vi "1.Main demo.vi"() -> ()   [LabVIEW 2015]
uses:
  UnderAutomation.Fanuc/UnderAutomation.Fanuc.lvlib
  C:/Users/fg/Documents/Fanuc.vi/LabVIEW_2024/UnderAutomation.Fanuc/lib/UnderAutomation.Fanuc.dll
  LabVIEW_2024/UnderAutomation.Fanuc/lib/UnderAutomation.Fanuc.dll
panel:
  out "CGTP Enabled":bool
  out "Cgtp":refnum<k24>
  out "SNPX connected":bool
  out "FTP connected":bool
  out "Telnet connected":bool
  in  "Tab Control":T1(tab)
  in  "HTTP Password":string caption="HTTP password"
  in  "HTTP Login":string caption="HTTP login (optional)"
  in  "Use CGTP":bool
  in  "Disconnect":bool
  in  "Test":bool
  in  "Key":string
  in  "Licensee":string
  in  "Use SNPX":bool
  in  "FTP password":string
  in  "FTP user":string
  in  "Use FTP":bool
  in  "Connect":bool
  in  "Telnet password":string
  in  "Use Telnet":bool
  in  "ConnectRoboguide":bool
  in  "RoboguideRobotPath":path caption="Path to \"Robot\" ROBOGUIDE folder that contains services.txt"
  in  "IP":string caption="Robot IP Address"
  out "License state":string
  out "Connect error":string
  out "CGTP warning":string
  in  "Abort":bool
  in  "Pause":bool
  in  "Program name":string caption="Program name without extension"
  in  "Run":bool
  in  "Write variable as real":bool
  in  "New integer value":i32
  in  "New real value":dbl
  in  "String value":string
  in  "Variable name":string
  in  "Write variable as integer":bool
  in  "Read variable":bool
  in  "Write variable as string":bool
  in  "Unsimulate all":bool
  in  "Unsimulate":bool
  in  "Simulate":bool
  in  "Set port value":bool
  in  "Variable set value":bool
  in  "Variable new value":string caption="New value"
  in  "Variable get value":bool
  in  "Variable name":string
  out "Telnet warning":string
  out "Current position":T2
  in  "Get current position":bool
  in  "Reset alarms":bool
  in  "Get task info":bool
  in  "Task name":string caption="Task name (program without extension)"
  in  "Abort all programs":bool
  in  "Clear variable":bool
  in  "Clear Program":bool
  in  "Hold":bool
  in  "Continue":bool
  in  "Abort":bool
  in  "Pause":bool
  in  "Program name":string caption="Program name without extension"
  in  "Run":bool
  out "TelnetError":string caption="Error :"
  out "TelnetSucceed":bool caption="Succeeded"
  out "KclCommand":string caption="Last command :"
  out "TaskInfo":T3
  out "Variable value":string
  in  "port":i32(ring) items=["DIN", "DOUT", "RDO", "OPOUT", "TPOUT", "WDI", "WDO", "AIN", "AOUT", "GIN", "GOUT"]
  in  "index":i32
  in  "value":i32
  out "FTP warning":string
  out "PosReg":T4(array[cluster])
  out "StrReg":string[](array[string])
  in  "Tab Control IO state":T5(tab)
  out "UI":cluster{"Id":i32, "Name":string, "Value":bool}[](array[cluster])
  out "UO":cluster{"Id":i32, "Name":string, "Value":bool}[](array[cluster])
  out "SI":cluster{"Id":i32, "Name":string, "Value":bool}[](array[cluster])
  out "SO":cluster{"Id":i32, "Name":string, "Value":bool}[](array[cluster])
  out "DIN":cluster{"Id":i32, "Name":string, "Value":bool}[](array[cluster])
  out "DOUT":cluster{"Id":i32, "Name":string, "Value":bool}[](array[cluster])
  out "RI":cluster{"Id":i32, "Name":string, "Value":bool}[](array[cluster])
  out "RO":cluster{"Id":i32, "Name":string, "Value":bool}[](array[cluster])
  out "FLG":cluster{"Id":i32, "Name":string, "Value":bool}[](array[cluster])
  in  "Tab Control position":enum32{"World", "Joints", "User frames"}(tab)
  out "World Positions":T6(array[cluster])
  out "JointsPosition":dbl[](array[numeric])
  out "UserFramePositions":T7(array[cluster])
  in  "Get current position":bool
  in  "Get IO State":bool
  in  "Port":i32(ring) items=["DIN", "DOUT", "UI", "UO", "SI", "SO", "RI", "RO", "FLG"]
  out "Errors":T8(array[cluster])
  in  "Get all errors":bool
  in  "Get safety status":bool
  out "SafetyStatus":T9
  out "NumReg":dbl[](array[numeric])
  in  "Get numeric registers":bool
  in  "Get string registers":bool
  in  "Get position registers":bool
  out "SNPX warning":string
  in  "Tab Control snpx register":enum32{"Cartesian", "Joints"}(tab)
  in  "Cartesian position 2":T10
  in  "Write cartesian position register":bool
  in  "Joints position":dbl[](array[numeric])
  in  "Write joints position register":bool
  in  "Position register":i32
  in  "Read position register":bool
  out "Value":string
  in  "New value":string
  in  "String register":i32
  in  "Read string register":bool
  in  "Write string register":bool
  in  "Continuous read world position":bool
  out "JointsPosition":dbl[](array[numeric])
  out "Cartesian position":T11
  out "UserTool":i16
  out "error out":errorcluster
  in  "Continuous read user frame position":bool
  in  "userFrame":i32
  out "Cartesian position":T11
  out "UserTool":i16
  out "error out 2":errorcluster
  in  "Numeric register":i32
  in  "New value":sgl
  out "Value":sgl
  in  "Read numeric register":bool
  in  "Write numeric register":bool
  out "UserFrame":i16
  out "UserTool":i16
  in  "stop":bool
  out "Snpx":refnum<k24>
  out "Ftp":refnum<k24>
  out "Telnet":refnum<k24>
  out "robot":refnum<k24>
  # "UnderAutomation"
  # "https://underautomation.com/fanuc"
  # "+"
  # "LabVIEW demo app for remote control and monitoring of your Fanuc robot"
  # "Connect to robot"
  # "2. Ensure you have a trial or lifetime valid license"
  # "1. Set Fanuc robot address"
  # "This is a commercial library, you have a 30-day trial period. But you can use it forever if you buy a perpetual licence for your company (regardless of the number of robot, applications or developers)."
  # "Connect to real robot"
  # "Connect to ROBOGUIDE"
  # "If you have a license :"
  # "3. Select the services you want to connect to"
  # "CGTP"
  # "Telnet"
  # "FTP"
  # "SNPX"
  # "You need option R553 \"HMI Device SNPX\" \nor R651 FRL"
  # "How to enable Telnet : https://underautomation.com/fanuc/documentation/enable-telnet"
  # "See : https://underautomation.com/fanuc/documentation/snpx"
  # "4. Connect to the robot"
  # "CGTP"
  # "Please note that other CGTP features are available and can be provided upon request. Please contact UnderAutomation."
  # "Program execution"
  # "Variable"
  # "Telnet"
  # "Variables"
  # "Program execution"
  # "Task"
  # "Ports"
  # "Current position"
  # "Alarms"
  # "FTP"
  # "Current Position"
  # "IO State"
  # "Errors"
  # "Registers"
  # "Safety status"
  # "SNPX"
  # "Numeric registers"
  # "String registers"
  # "Read world position"
  # "Read user frame position"
  # "Position registers"
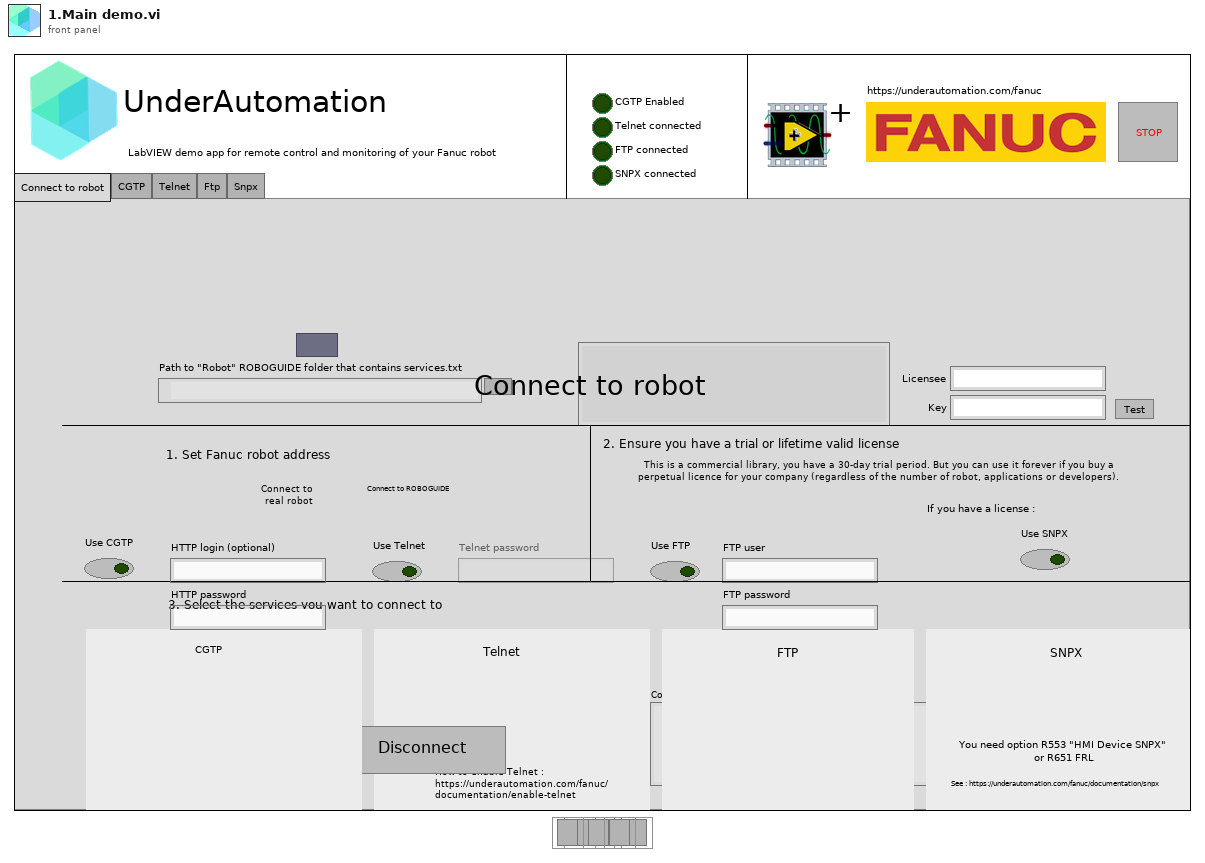
[diagram p1: front panel]
types:
  T1 = enum32{"Connect to robot", "CGTP", "Telnet", "Ftp", "Snpx"}
  T2 = cluster{"X":dbl, "Y":dbl, "Z":dbl, "W":dbl, "P":dbl, "R":dbl}
  T3 = cluster{"CurrentLine":i32, "RoutineName":string, "SystemTask":bool, "TaskName":string, "TaskNumber":i32, "TaskStatus":i32, "TaskStatusStr":string}
  T4 = cluster{"X":dbl, "Y":dbl, "Z":dbl, "W":dbl, "P":dbl, "R":dbl}[][]
  T5 = enum32{"UI", "UO", "SI", "SO", "DIN", "DOUT", "RI", "RO", "FLG"}
  T6 = cluster{"Tool":i32, "Cartesian position":cluster{cluster{"ArmFrontBack":i32, "ArmLeftRight":i32, "ArmUpDown":i32, "TurnAxis1":i32, "TurnAxis2":i32, "TurnAxis3":i32, "WristFlip":i32}, "X":dbl, "Y":dbl, "Z":dbl, "W":dbl, "P":dbl, "R":dbl}}[]
  T7 = cluster{"Frame":i32, "Tool":i32, "Cartesian position":cluster{cluster{"ArmFrontBack":i32, "ArmLeftRight":i32, "ArmUpDown":i32, "TurnAxis1":i32, "TurnAxis2":i32, "TurnAxis3":i32, "WristFlip":i32}, "X":dbl, "Y":dbl, "Z":dbl, "W":dbl, "P":dbl, "R":dbl}}[]
  T8 = cluster{"Id":i32, "IsReset":bool, "Text":string}[]
  T9 = cluster{"BeltBroken":bool, "ExternalEStop":bool, "FenceOpen":bool, "HandBroken":bool, "LowAirAlarm":bool, "NonTeacherEnb":bool, "OverTravel":bool, "SOPEStop":bool, "SVOFFDetect":bool, "TPDeadman":bool, "TPEnable":bool, "TPEStop":bool}
  T10 = cluster{"Configuration":cluster{"ArmFrontBack":i32, "ArmLeftRight":i32, "ArmUpDown":i32, "TurnAxis1":i32, "TurnAxis2":i32, "TurnAxis3":i32, "WristFlip":i32}, "X":dbl, "Y":dbl, "Z":dbl, "W":dbl, "P":dbl, "R":dbl}
  T11 = cluster{"Cartesian position":cluster{cluster{"ArmFrontBack":i32, "ArmLeftRight":i32, "ArmUpDown":i32, "TurnAxis1":i32, "TurnAxis2":i32, "TurnAxis3":i32, "WristFlip":i32}, "X":dbl, "Y":dbl, "Z":dbl, "W":dbl, "P":dbl, "R":dbl}, "Extension":cluster{"E1":dbl, "E2":dbl, "E3":dbl, "T4":i16, "T5":i16, "T6":i16}}
  T12 = enum8{"Enabled", "Disabled", "Disabled and Grayed Out"}
  T13 = cluster{"Id":i32, "Values":dbl[], "UserFramePositions":cluster{"Frame":i32, "Tool":i32, "Cartesian position":cluster{cluster{"ArmFrontBack":i32, "ArmLeftRight":i32, "ArmUpDown":i32, "TurnAxis1":i32, "TurnAxis2":i32, "TurnAxis3":i32, "WristFlip":i32}, "X":dbl, "Y":dbl, "Z":dbl, "W":dbl, "P":dbl, "R":dbl}}[], "World Positions":cluster{"Tool":i32, "Cartesian position":cluster{cluster{"ArmFrontBack":i32, "ArmLeftRight":i32, "ArmUpDown":i32, "TurnAxis1":i32, "TurnAxis2":i32, "TurnAxis3":i32, "WristFlip":i32}, "X":dbl, "Y":dbl, "Z":dbl, "W":dbl, "P":dbl, "R":dbl}}[]}[]
  T14 = cluster{"Id":i32, "Name":string, "Port":i32, "Value":bool, "PortStr":string}[]
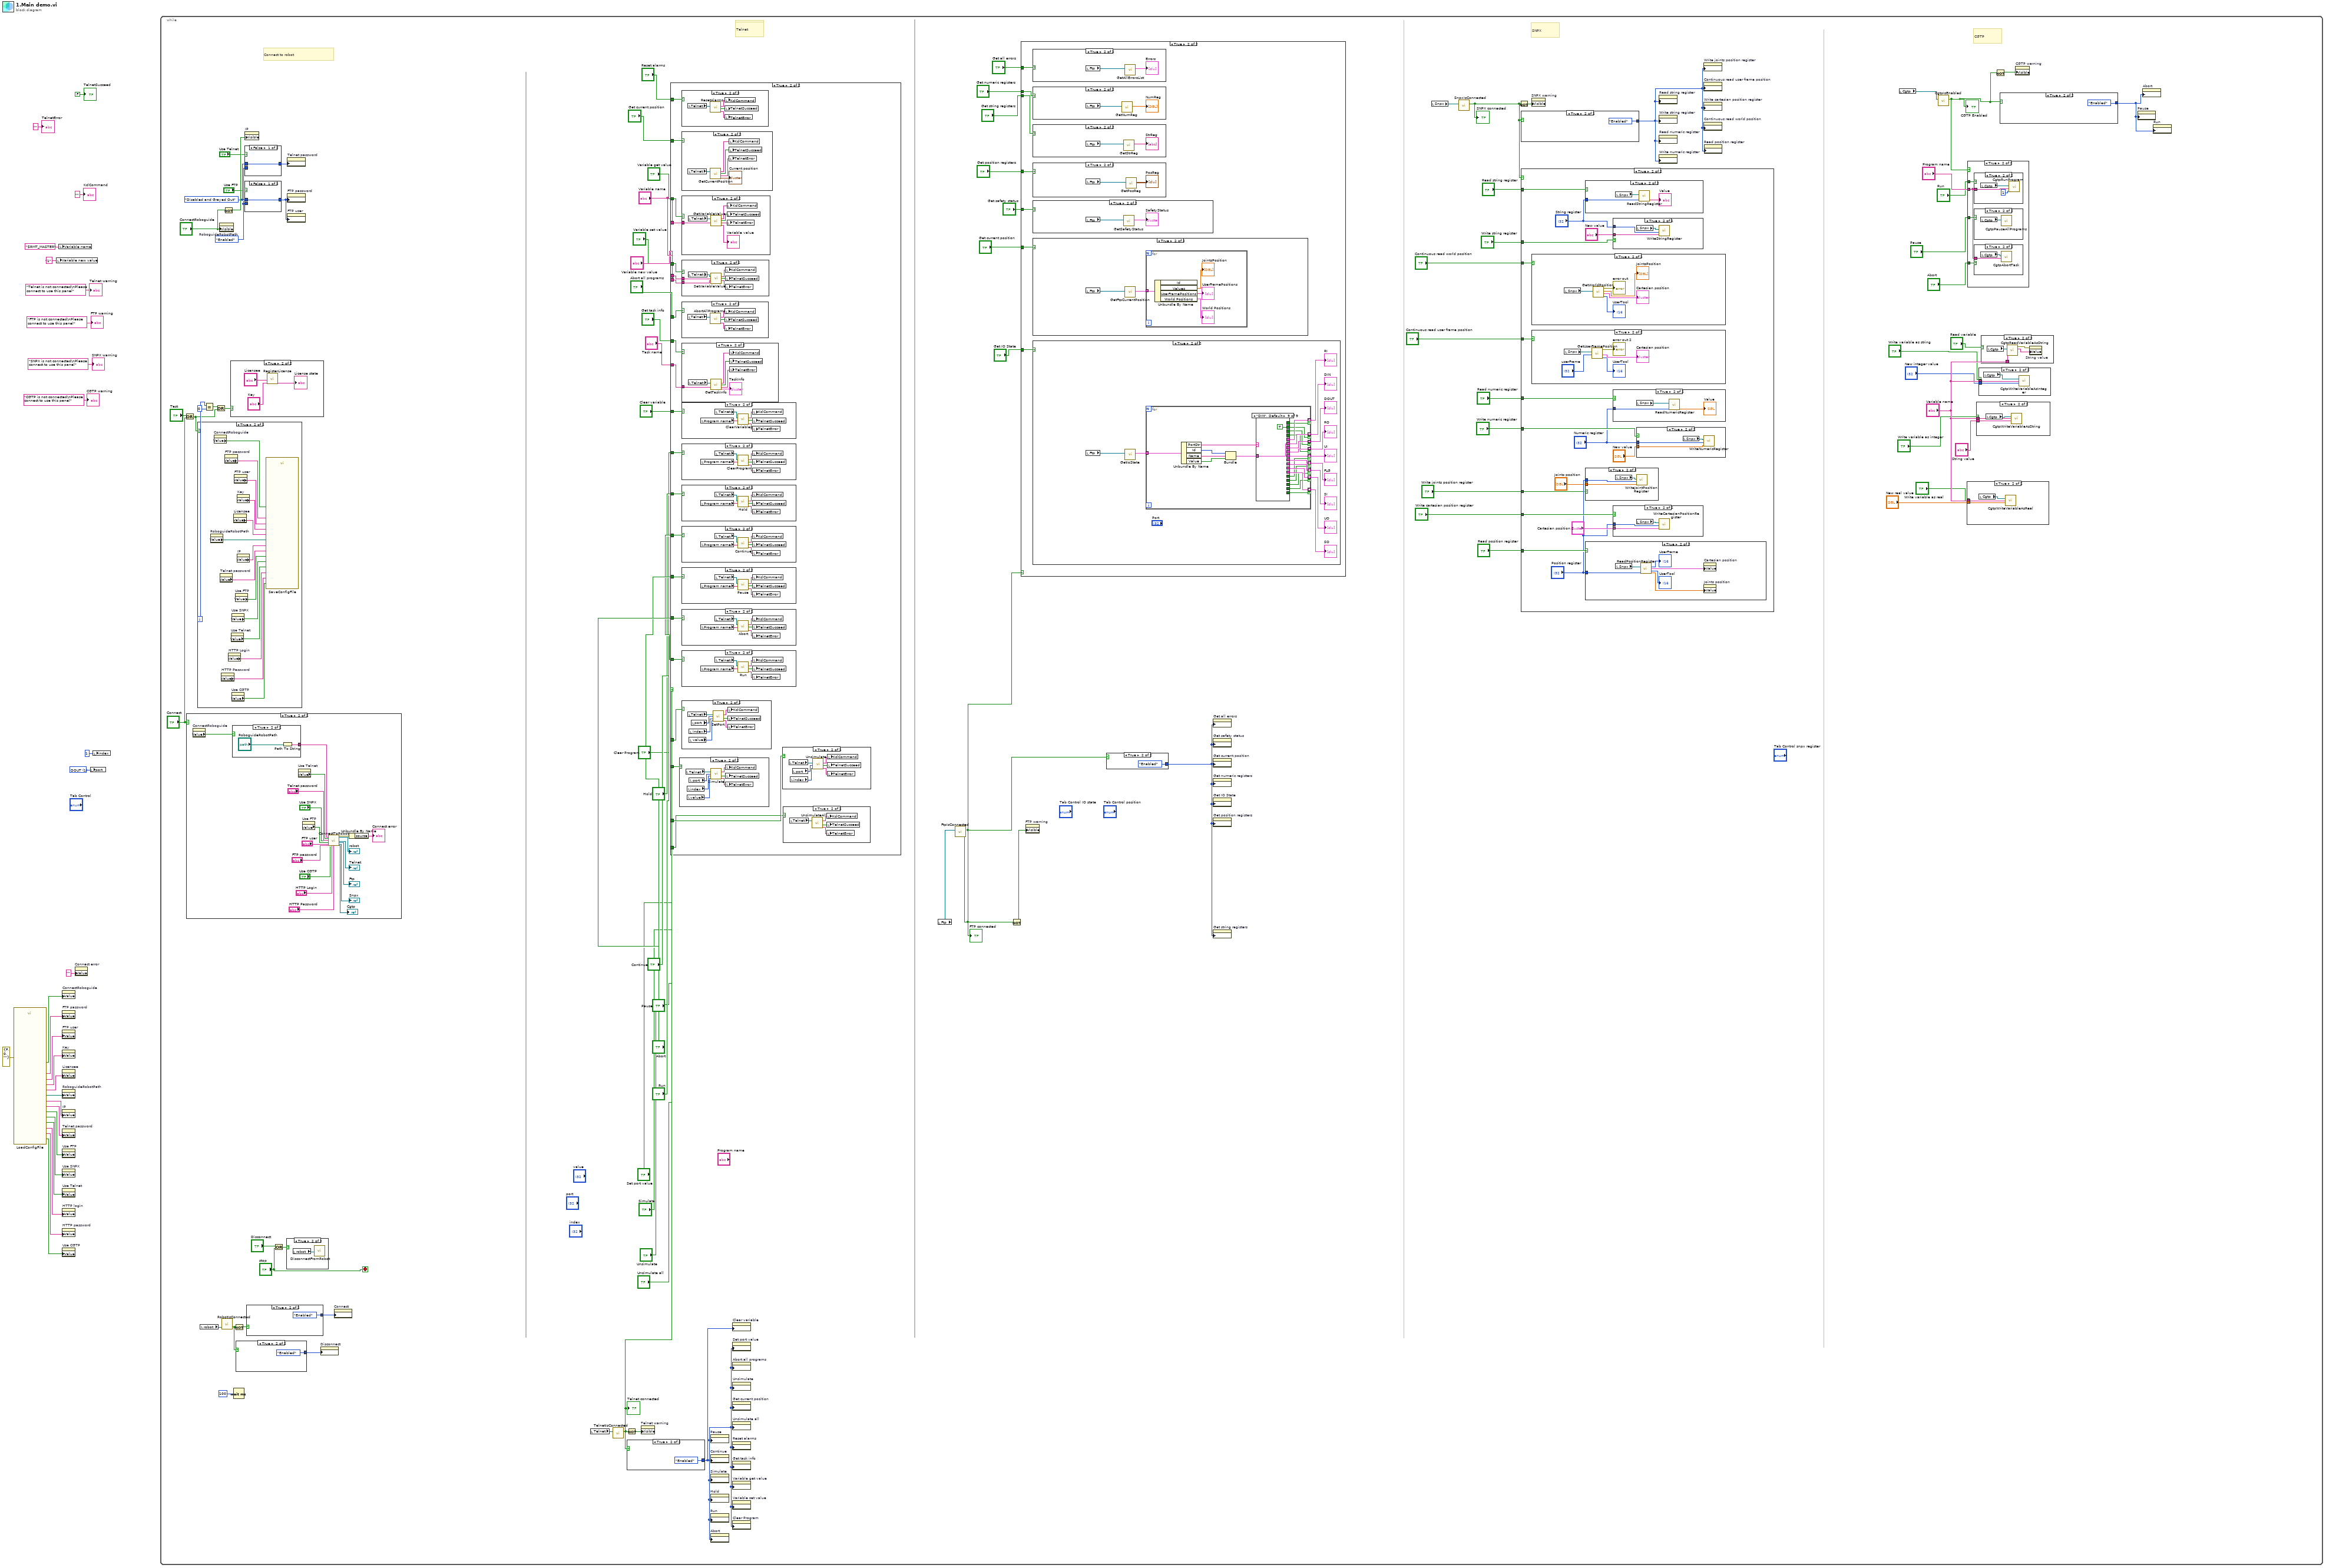
[diagram p0: block diagram]
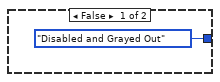
[diagram p10: hidden frame]
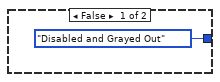
[diagram p11: hidden frame]
diagram:
  w7 = 1 items=["DIN", "DOUT", "RDO", "OPOUT", "TPOUT", "WDI", "WDO", "AIN", "AOUT", "GIN", "GOUT"] ("port")
  n1 = call "LoadConfigFile.vi"("error in (no error)"=errorcluster {"status"=FALSE, "code"=0, "source"=""}) -> ("Use CGTP"=w2:bool, "HTTP login"=w3:string, "HTTP password"=w4:string, "FTP password"=w24:string, "Licensee"=w16:string, "FTP user"=w23:string, "Key"=w17:string, "Use FTP"=w20:bool, "IP"=w26:string, "RoboguideRobotPath"=w22:path, "ConnectRoboguide"=w25:bool, "Use Telnet"=w18:bool, "Telnet password"=w21:string, "Use SNPX"=w19:bool)  [unwired: 12 in, 1 out]
  n2 = local write "Variable new value"("1" ("Variable new value")) -> ()
  n3 = local write "Variable name"("$RMT_MASTER" ("Variable name")) -> ()
  n4 = property on="ConnectRoboguide" class="Bool (strict)"("Value"=w25) -> ()  [unwired: 2 in, 2 out]
  n5 = property on="FTP password" class="Str"("Value"=w24) -> ()  [unwired: 2 in, 2 out]
  n6 = property on="FTP user" class="Str"("Value"=w23) -> ()  [unwired: 2 in, 2 out]
  n7 = property on="Key" class="Str"("Value"=w17) -> ()  [unwired: 2 in, 2 out]
  n8 = property on="Licensee" class="Str"("Value"=w16) -> ()  [unwired: 2 in, 2 out]
  n9 = property on="RoboguideRobotPath" class="Path"("Value"=w22) -> ()  [unwired: 2 in, 2 out]
  n10 = property on="IP" class="Str"("Value"=w26) -> ()  [unwired: 2 in, 2 out]
  n11 = property on="Telnet password" class="Str"("Value"=w21) -> ()  [unwired: 2 in, 2 out]
  n12 = property on="Use FTP" class="Bool (strict)"("Value"=w20) -> ()  [unwired: 2 in, 2 out]
  n13 = property on="Use SNPX" class="Bool (strict)"("Value"=w19) -> ()  [unwired: 2 in, 2 out]
  n14 = property on="Use Telnet" class="Bool (strict)"("Value"=w18) -> ()  [unwired: 2 in, 2 out]
  n15 = property on="HTTP login" class="Str"("Value"=w3) -> ()  [unwired: 2 in, 2 out]
  n16 = property on="HTTP password" class="Str"("Value"=w4) -> ()  [unwired: 2 in, 2 out]
  n17 = property on="Use CGTP" class="Bool (strict)"("Value"=w2) -> ()  [unwired: 2 in, 2 out]
  n18 = property on="Connect error" class="Str"("Value"="" ("Connect error")) -> ()  [unwired: 2 in, 2 out]
  n19 = local write "port"(w7) -> ()
  n20 = local write "index"(1 ("index")) -> ()
  n21 = while {
    i -> [w110]
    stop <- "stop" stop-if-true
    w102 = T12."Enabled" ("Disabled")
    w103 = T12."Disabled and Grayed Out" ("Disabled")
    # "CGTP"
    # "SNPX"
    # "FTP"
    # "Telnet"
    # "Connect to robot"
    n22 = Or(x="Test", y="Connect") -> (x .or. y?=w107:bool)
    n23 = case shown="True" "Connect" {
      frame False {
      }
      frame True {
        n24 = property on="ConnectRoboguide" class="Bool (strict)"() -> ("Value"=w427:bool)  [unwired: 2 in, 2 out]
        n25 = case shown="True" w427 {
          tunnel: ["IP" w429] -> w426
          frame False {
          }
          frame True {
            n26 = Path To String(path="RoboguideRobotPath") -> (string=w429:string)
          }
        }
        n27 = property on="Use Telnet" class="Bool (strict)"() -> ("Value"=w422:bool)  [unwired: 2 in, 2 out]
        n28 = property on="Use FTP" class="Bool (strict)"() -> ("Value"=w421:bool)  [unwired: 2 in, 2 out]
        n29 = call "ConnectToRobot.vi"("address"=w426, "Telnet enable"=w422, "Telnet KCL password"="Telnet password", "SNPX enable"="Use SNPX", "FTP enable"=w421, "FTP user"="FTP user", "FTP password"="FTP password", "CGTP enable"="Use CGTP", "HTTP login"="HTTP Login", "HTTP password"="HTTP Password") -> ("error out"=w420:errorcluster, "robot"=→"robot":refnum<k24>, "Telnet"=→"Telnet":refnum<k24>, "Ftp"=→"Ftp":refnum<k24>, "Snpx"=→"Snpx":refnum<k24>, "Cgtp"=→"Cgtp":refnum<k24>)  [unwired: 12 in]
        n30 = Unbundle By Name(w420) -> ("source"=→"Connect error":string)
      }
    }
    n31 = case shown="True" w107 {
      frame False {
      }
      frame True {
        n32 = property on="RoboguideRobotPath" class="Path"() -> ("Value"=w404:path)  [unwired: 2 in, 2 out]
        n33 = property on="ConnectRoboguide" class="Bool (strict)"() -> ("Value"=w409:bool)  [unwired: 2 in, 2 out]
        n34 = property on="Telnet password" class="Str"() -> ("Value"=w402:string)  [unwired: 2 in, 2 out]
        n35 = property on="HTTP Password" class="Str"() -> ("Value"=w396:string)  [unwired: 2 in, 2 out]
        n36 = property on="FTP password" class="Str"() -> ("Value"=w408:string)  [unwired: 2 in, 2 out]
        n37 = property on="HTTP Login" class="Str"() -> ("Value"=w397:string)  [unwired: 2 in, 2 out]
        n38 = property on="Use Telnet" class="Bool (strict)"() -> ("Value"=w399:bool)  [unwired: 2 in, 2 out]
        n39 = property on="Use SNPX" class="Bool (strict)"() -> ("Value"=w400:bool)  [unwired: 2 in, 2 out]
        n40 = property on="Use CGTP" class="Bool (strict)"() -> ("Value"=w398:bool)  [unwired: 2 in, 2 out]
        n41 = property on="Licensee" class="Str"() -> ("Value"=w405:string)  [unwired: 2 in, 2 out]
        n42 = property on="FTP user" class="Str"() -> ("Value"=w407:string)  [unwired: 2 in, 2 out]
        n43 = property on="Use FTP" class="Bool (strict)"() -> ("Value"=w401:bool)  [unwired: 2 in, 2 out]
        n44 = property on="Key" class="Str"() -> ("Value"=w406:string)  [unwired: 2 in, 2 out]
        n45 = property on="IP" class="Str"() -> ("Value"=w403:string)  [unwired: 2 in, 2 out]
        n46 = call "SaveConfigFile.vi"("IP"=w403, "RoboguideRobotPath"=w404, "ConnectRoboguide"=w409, "Use Telnet"=w399, "Telnet password"=w402, "Use FTP"=w401, "FTP user"=w407, "FTP password"=w408, "Use SNPX"=w400, "Licensee"=w405, "Use CGTP"=w398, "Key"=w406, "HTTP Login"=w397, "HTTP Password"=w396) -> ()  [unwired: 14 in]
      }
    }
    n47 = local read "robot"() -> (w77:refnum<k24>)
    n48 = Equal?(x=w110, y=0) -> (x = y?=w108:bool)
    n49 = Or(x=w108, y=w107) -> (x .or. y?=w106:bool)
    n50 = property on="RoboguideRobotPath" class="Path"("Visible"="ConnectRoboguide") -> ()  [unwired: 2 in, 2 out]
    n51 = call "RobotIsConnected.vi"("robot"=w77) -> ("Connected"=w75:bool)  [unwired: 1 in, 1 out]
    n52 = Not(x="ConnectRoboguide") -> (.not. x?=w114:bool)
    n53 = case shown="True" w106 {
      frame False {
      }
      frame True {
        n54 = call "RegisterLicense.vi"("key"="Key", "licensee"="Licensee") -> ("status"=→"License state":string)  [unwired: 7 in, 2 out]
      }
    }
    n55 = Wait (ms)(milliseconds to wait=u32 100) -> ()  [unwired: 1 out]
    n56 = Not(x=w75) -> (.not. x?=w76:bool)
    n57 = case shown="True" w75 {
      tunnel: [T12."Disabled and Grayed Out" ("Disabled") T12."Enabled" ("Disabled")] -> w74
      frame False {
      }
      frame True {
      }
    }
    n58 = property on="IP" class="Str"("Visible"=w114) -> ()  [unwired: 2 in, 2 out]
    n59 = case shown="False" "Use Telnet" {
      tunnel: w102 -> [_ w392]
      tunnel: [w391 w392] -> w104
      tunnel: w103 -> [w391 _]
      frame False {
      }
      frame True {
      }
    }
    n60 = case shown="False" "Use FTP" {
      tunnel: w102 -> [_ w390]
      tunnel: [w389 w390] -> w100
      tunnel: w103 -> [w389 _]
      frame False {
      }
      frame True {
      }
    }
    n61 = case shown="True" w76 {
      tunnel: [T12."Disabled and Grayed Out" ("Disabled") T12."Enabled" ("Disabled")] -> w73
      frame False {
      }
      frame True {
      }
    }
    n62 = Or(x="Disconnect", y="stop") -> (x .or. y?=w79:bool)
    n63 = case shown="True" w79 {
      frame False {
      }
      frame True {
        n64 = local read "robot"() -> (w275:refnum<k24>)
        n65 = call "DisconnectFromRobot.vi"("robot"=w275) -> ()  [unwired: 26 in, 1 out]
      }
    }
    n66 = property on="Telnet password" class="Str"("DisabledEnum"=w104) -> ()  [unwired: 2 in, 2 out]
    n67 = property on="FTP password" class="Str"("DisabledEnum"=w100) -> ()  [unwired: 2 in, 2 out]
    n68 = property on="FTP user" class="Str"("DisabledEnum"=w100) -> ()  [unwired: 2 in, 2 out]
    n69 = property on="Disconnect" class="Bool"("DisabledEnum"=w74) -> ()  [unwired: 2 in, 2 out]
    n70 = property on="Connect" class="Bool"("DisabledEnum"=w73) -> ()  [unwired: 2 in, 2 out]
    n71 = local read "Telnet"() -> (w99:refnum<k24>)
    n72 = call "TelnetIsConnected.vi"("Telnet"=w99) -> ("Connected"=w97:bool)  [unwired: 9 in, 1 out]
    "Telnet connected" <- w97
    n73 = Not(x=w97) -> (.not. x?=w96:bool)
    n74 = case shown="True" w97 {
      tunnel: [T12."Disabled and Grayed Out" ("Disabled") T12."Enabled" ("Disabled")] -> w68
      frame False {
      }
      frame True {
      }
    }
    n75 = property on="Telnet warning" class="Str"("Visible"=w96) -> ()  [unwired: 2 in, 2 out]
    n76 = case shown="True" w97 {
      tunnel: "Run" -> [_ w298]
      tunnel: "Abort" -> [_ w297]
      tunnel: "Pause" -> [_ w296]
      tunnel: "Continue" -> [_ w295]
      tunnel: "Hold" -> [_ w294]
      tunnel: "Clear variable" -> [_ w293]
      tunnel: "Clear Program" -> [_ w292]
      tunnel: "Abort all programs" -> [_ w291]
      tunnel: "Task name" -> [_ w290]
      tunnel: "Get task info" -> [_ w289]
      tunnel: "Reset alarms" -> [_ w288]
      tunnel: "Get current position" -> [_ w287]
      tunnel: "Variable get value" -> [_ w286]
      tunnel: "Variable name" -> [_ w285]
      tunnel: "Variable name" -> [_ w284]
      tunnel: "Variable new value" -> [_ w283]
      tunnel: "Variable set value" -> [_ w282]
      tunnel: "Set port value" -> [_ w281]
      tunnel: "Simulate" -> [_ w280]
      tunnel: "Unsimulate" -> [_ w279]
      tunnel: "Unsimulate all" -> [_ w278]
      frame False {
      }
      frame True {
        n77 = case shown="True" w280 {
          frame False {
          }
          frame True {
            n78 = local read "Telnet"() -> (w312:refnum<k24>)
            n79 = local read "index"() -> (w309:i32)
            n80 = local read "value"() -> (w311:i32)
            n81 = local read "port"() -> (w310:i32)
            n82 = call "Simulate.vi"("Telnet"=w312, "port"=w310, "index"=w309, "value"=w311) -> ("KclCommand"=w315:string, "Succeed"=w314:bool, "ErrorText"=w313:string)  [unwired: 8 in, 1 out]
            n83 = local write "KclCommand"(w315) -> ()
            n84 = local write "TelnetSucceed"(w314) -> ()
            n85 = local write "TelnetError"(w313) -> ()
          }
        }
        n86 = case shown="True" w288 {
          frame False {
          }
          frame True {
            n87 = local read "Telnet"() -> (w343:refnum<k24>)
            n88 = call "ResetAlarms.vi"("Telnet"=w343) -> ("ErrorText"=w341:string, "Succeed"=w342:bool, "KclCommand"=w340:string)  [unwired: 7 in, 1 out]
            n89 = local write "KclCommand"(w340) -> ()
            n90 = local write "TelnetSucceed"(w342) -> ()
            n91 = local write "TelnetError"(w341) -> ()
          }
        }
        n92 = case shown="True" w287 {
          frame False {
          }
          frame True {
            n93 = local read "Telnet"() -> (w339:refnum<k24>)
            n94 = call "GetCurrentPosition.vi"("Telnet"=w339) -> ("KclCommand"=w337:string, "Succeed"=w336:bool, "ErrorText"=w335:string, "Position"=→"Current position":T2)  [unwired: 10 in, 1 out]
            n95 = local write "KclCommand"(w337) -> ()
            n96 = local write "TelnetSucceed"(w336) -> ()
            n97 = local write "TelnetError"(w335) -> ()
          }
        }
        n98 = case shown="True" w286 {
          tunnel: w285 -> [_ w333]
          frame False {
          }
          frame True {
            n99 = local read "Telnet"() -> (w334:refnum<k24>)
            n100 = call "GetVariableValue.vi"("Telnet"=w334, "name"=w333) -> ("KclCommand"=w329:string, "Succeed"=w330:bool, "ErrorText"=w331:string, "RawValue"=→"Variable value":string)  [unwired: 9 in, 1 out]
            n101 = local write "KclCommand"(w329) -> ()
            n102 = local write "TelnetSucceed"(w330) -> ()
            n103 = local write "TelnetError"(w331) -> ()
          }
        }
        n104 = case shown="True" w282 {
          tunnel: w284 -> [_ w327]
          tunnel: w283 -> [_ w326]
          frame False {
          }
          frame True {
            n105 = local read "Telnet"() -> (w328:refnum<k24>)
            n106 = call "SetVariableValue.vi"("Telnet"=w328, "value"=w326, "name"=w327) -> ("KclCommand"=w325:string, "Succeed"=w324:bool, "ErrorText"=w323:string)  [unwired: 9 in, 1 out]
            n107 = local write "KclCommand"(w325) -> ()
            n108 = local write "TelnetSucceed"(w324) -> ()
            n109 = local write "TelnetError"(w323) -> ()
          }
        }
        n110 = case shown="True" w291 {
          frame False {
          }
          frame True {
            n111 = local read "Telnet"() -> (w350:refnum<k24>)
            n112 = call "AbortAllPrograms.vi"("Telnet"=w350) -> ("ErrorText"=w351:string, "Succeed"=w352:bool, "KclCommand"=w353:string)  [unwired: 7 in, 1 out]
            n113 = local write "KclCommand"(w353) -> ()
            n114 = local write "TelnetSucceed"(w352) -> ()
            n115 = local write "TelnetError"(w351) -> ()
          }
        }
        n116 = case shown="True" w289 {
          tunnel: w290 -> [_ w348]
          frame False {
          }
          frame True {
            n117 = local read "Telnet"() -> (w349:refnum<k24>)
            n118 = call "GetTaskInfo.vi"("Telnet"=w349, "task"=w348) -> ("KclCommand"=w346:string, "Succeed"=w345:bool, "ErrorText"=w344:string, "TaskInfo"=→"TaskInfo":T3)  [unwired: 9 in, 1 out]
            n119 = local write "KclCommand"(w346) -> ()
            n120 = local write "TelnetSucceed"(w345) -> ()
            n121 = local write "TelnetError"(w344) -> ()
          }
        }
        n122 = case shown="True" w293 {
          frame False {
          }
          frame True {
            n123 = local read "Program name"() -> (w354:string)
            n124 = local read "Telnet"() -> (w355:refnum<k24>)
            n125 = call "ClearVariables.vi"("program"=w354, "Telnet"=w355) -> ("ErrorText"=w356:string, "Succeed"=w357:bool, "KclCommand"=w358:string)  [unwired: 6 in, 1 out]
            n126 = local write "KclCommand"(w358) -> ()
            n127 = local write "TelnetSucceed"(w357) -> ()
            n128 = local write "TelnetError"(w356) -> ()
          }
        }
        n129 = case shown="True" w292 {
          frame False {
          }
          frame True {
            n130 = local read "Program name"() -> (w359:string)
            n131 = local read "Telnet"() -> (w360:refnum<k24>)
            n132 = call "ClearProgram.vi"("program"=w359, "Telnet"=w360) -> ("ErrorText"=w361:string, "Succeed"=w362:bool, "KclCommand"=w363:string)  [unwired: 6 in, 1 out]
            n133 = local write "KclCommand"(w363) -> ()
            n134 = local write "TelnetSucceed"(w362) -> ()
            n135 = local write "TelnetError"(w361) -> ()
          }
        }
        n136 = case shown="True" w294 {
          frame False {
          }
          frame True {
            n137 = local read "Program name"() -> (w364:string)
            n138 = local read "Telnet"() -> (w365:refnum<k24>)
            n139 = call "Hold.vi"("program"=w364, "Telnet"=w365) -> ("ErrorText"=w366:string, "Succeed"=w367:bool, "KclCommand"=w368:string)  [unwired: 6 in, 1 out]
            n140 = local write "KclCommand"(w368) -> ()
            n141 = local write "TelnetSucceed"(w367) -> ()
            n142 = local write "TelnetError"(w366) -> ()
          }
        }
        n143 = case shown="True" w295 {
          frame False {
          }
          frame True {
            n144 = local read "Program name"() -> (w369:string)
            n145 = local read "Telnet"() -> (w370:refnum<k24>)
            n146 = call "Continue.vi"("program"=w369, "Telnet"=w370) -> ("ErrorText"=w371:string, "Succeed"=w372:bool, "KclCommand"=w373:string)  [unwired: 6 in, 1 out]
            n147 = local write "KclCommand"(w373) -> ()
            n148 = local write "TelnetSucceed"(w372) -> ()
            n149 = local write "TelnetError"(w371) -> ()
          }
        }
        n150 = case shown="True" w296 {
          frame False {
          }
          frame True {
            n151 = local read "Program name"() -> (w374:string)
            n152 = local read "Telnet"() -> (w375:refnum<k24>)
            n153 = call "Pause.vi"("program"=w374, "Telnet"=w375) -> ("ErrorText"=w376:string, "Succeed"=w377:bool, "KclCommand"=w378:string)  [unwired: 6 in, 1 out]
            n154 = local write "KclCommand"(w378) -> ()
            n155 = local write "TelnetSucceed"(w377) -> ()
            n156 = local write "TelnetError"(w376) -> ()
          }
        }
        n157 = case shown="True" w297 {
          frame False {
          }
          frame True {
            n158 = local read "Program name"() -> (w379:string)
            n159 = local read "Telnet"() -> (w380:refnum<k24>)
            n160 = call "Abort.vi"("program"=w379, "Telnet"=w380) -> ("ErrorText"=w381:string, "Succeed"=w382:bool, "KclCommand"=w383:string)  [unwired: 6 in, 1 out]
            n161 = local write "KclCommand"(w383) -> ()
            n162 = local write "TelnetSucceed"(w382) -> ()
            n163 = local write "TelnetError"(w381) -> ()
          }
        }
        n164 = case shown="True" w298 {
          frame False {
          }
          frame True {
            n165 = local read "Program name"() -> (w384:string)
            n166 = local read "Telnet"() -> (w385:refnum<k24>)
            n167 = call "Run.vi"("program"=w384, "Telnet"=w385) -> ("ErrorText"=w386:string, "Succeed"=w387:bool, "KclCommand"=w388:string)  [unwired: 6 in, 1 out]
            n168 = local write "KclCommand"(w388) -> ()
            n169 = local write "TelnetSucceed"(w387) -> ()
            n170 = local write "TelnetError"(w386) -> ()
          }
        }
        n171 = case shown="True" w281 {
          frame False {
          }
          frame True {
            n172 = local read "Telnet"() -> (w319:refnum<k24>)
            n173 = local read "index"() -> (w316:i32)
            n174 = local read "value"() -> (w318:i32)
            n175 = local read "port"() -> (w317:i32)
            n176 = call "SetPort.vi"("Telnet"=w319, "port"=w317, "index"=w316, "value"=w318) -> ("KclCommand"=w322:string, "Succeed"=w321:bool, "ErrorText"=w320:string)  [unwired: 8 in, 1 out]
            n177 = local write "KclCommand"(w322) -> ()
            n178 = local write "TelnetSucceed"(w321) -> ()
            n179 = local write "TelnetError"(w320) -> ()
          }
        }
        n180 = case shown="True" w279 {
          frame False {
          }
          frame True {
            n181 = local read "Telnet"() -> (w305:refnum<k24>)
            n182 = local read "index"() -> (w303:i32)
            n183 = local read "port"() -> (w304:i32)
            n184 = call "Unsimulate.vi"("index"=w303, "port"=w304, "Telnet"=w305) -> ("ErrorText"=w306:string, "Succeed"=w307:bool, "KclCommand"=w308:string)  [unwired: 5 in, 1 out]
            n185 = local write "KclCommand"(w308) -> ()
            n186 = local write "TelnetSucceed"(w307) -> ()
            n187 = local write "TelnetError"(w306) -> ()
          }
        }
        n188 = case shown="True" w278 {
          frame False {
          }
          frame True {
            n189 = local read "Telnet"() -> (w299:refnum<k24>)
            n190 = call "UnsimulateAll.vi"("Telnet"=w299) -> ("KclCommand"=w302:string, "Succeed"=w301:bool, "ErrorText"=w300:string)  [unwired: 11 in, 1 out]
            n191 = local write "KclCommand"(w302) -> ()
            n192 = local write "TelnetSucceed"(w301) -> ()
            n193 = local write "TelnetError"(w300) -> ()
          }
        }
      }
    }
    n194 = property on="Pause" class="Bool"("DisabledEnum"=w68) -> ()  [unwired: 2 in, 2 out]
    n195 = property on="Continue" class="Bool"("DisabledEnum"=w68) -> ()  [unwired: 2 in, 2 out]
    n196 = property on="Simulate" class="Bool"("DisabledEnum"=w68) -> ()  [unwired: 2 in, 2 out]
    n197 = property on="Hold" class="Bool"("DisabledEnum"=w68) -> ()  [unwired: 2 in, 2 out]
    n198 = property on="Run" class="Bool"("DisabledEnum"=w68) -> ()  [unwired: 2 in, 2 out]
    n199 = property on="Abort" class="Bool"("DisabledEnum"=w68) -> ()  [unwired: 2 in, 2 out]
    n200 = property on="Clear variable" class="Bool"("DisabledEnum"=w68) -> ()  [unwired: 2 in, 2 out]
    n201 = property on="Set port value" class="Bool"("DisabledEnum"=w68) -> ()  [unwired: 2 in, 2 out]
    n202 = property on="Abort all programs" class="Bool"("DisabledEnum"=w68) -> ()  [unwired: 2 in, 2 out]
    n203 = property on="Unsimulate" class="Bool"("DisabledEnum"=w68) -> ()  [unwired: 2 in, 2 out]
    n204 = property on="Get current position" class="Bool"("DisabledEnum"=w68) -> ()  [unwired: 2 in, 2 out]
    n205 = property on="Unsimulate all" class="Bool"("DisabledEnum"=w68) -> ()  [unwired: 2 in, 2 out]
    n206 = property on="Reset alarms" class="Bool"("DisabledEnum"=w68) -> ()  [unwired: 2 in, 2 out]
    n207 = property on="Get task info" class="Bool"("DisabledEnum"=w68) -> ()  [unwired: 2 in, 2 out]
    n208 = property on="Variable get value" class="Bool"("DisabledEnum"=w68) -> ()  [unwired: 2 in, 2 out]
    n209 = property on="Variable set value" class="Bool"("DisabledEnum"=w68) -> ()  [unwired: 2 in, 2 out]
    n210 = property on="Clear Program" class="Bool"("DisabledEnum"=w68) -> ()  [unwired: 2 in, 2 out]
    n211 = local read "Ftp"() -> (w67:refnum<k24>)
    n212 = call "FtpIsConnected.vi"("Ftp"=w67) -> ("Connected"=w58:bool)  [unwired: 9 in, 1 out]
    "FTP connected" <- w58
    n213 = Not(x=w58) -> (.not. x?=w59:bool)
    n214 = case shown="True" w58 {
      tunnel: "Get current position" -> [_ w201]
      tunnel: "Get IO State" -> [_ w200]
      tunnel: "Get all errors" -> [_ w199]
      tunnel: "Get safety status" -> [_ w198]
      tunnel: "Get numeric registers" -> [_ w197]
      tunnel: "Get string registers" -> [_ w196]
      tunnel: "Get position registers" -> [_ w195]
      frame False {
      }
      frame True {
        n215 = case shown="True" w199 {
          frame False {
          }
          frame True {
            n216 = local read "Ftp"() -> (w211:refnum<k24>)
            n217 = call "GetAllErrorsList.vi"("Ftp"=w211) -> ("Errors"=→"Errors":T8)  [unwired: 9 in, 1 out]
          }
        }
        n218 = case shown="True" w197 {
          frame False {
          }
          frame True {
            n219 = local read "Ftp"() -> (w207:refnum<k24>)
            n220 = call "GetNumReg.vi"("Ftp"=w207) -> ("NumReg"=→"NumReg":dbl[])  [unwired: 9 in, 1 out]
          }
        }
        n221 = case shown="True" w196 {
          frame False {
          }
          frame True {
            n222 = local read "Ftp"() -> (w205:refnum<k24>)
            n223 = call "GetStrReg.vi"("Ftp"=w205) -> ("StrReg"=→"StrReg":string[])  [unwired: 9 in, 1 out]
          }
        }
        n224 = case shown="True" w195 {
          frame False {
          }
          frame True {
            n225 = local read "Ftp"() -> (w203:refnum<k24>)
            n226 = call "GetPosReg.vi"("Ftp"=w203) -> ("PosReg"=→"PosReg":T4)  [unwired: 9 in, 1 out]
          }
        }
        n227 = case shown="True" w198 {
          frame False {
          }
          frame True {
            n228 = local read "Ftp"() -> (w209:refnum<k24>)
            n229 = call "GetSafetyStatus.vi"("Ftp"=w209) -> ("SafetyStatus"=→"SafetyStatus":T9)  [unwired: 9 in, 1 out]
          }
        }
        n230 = case shown="True" w201 {
          frame False {
          }
          frame True {
            n231 = local read "Ftp"() -> (w266:refnum<k24>)
            n232 = call "GetFtpCurrentPosition.vi"("Ftp"=w266) -> ("Current position"=w265:T13)  [unwired: 9 in, 1 out]
            n233 = for {
              tunnel: w265 -> [w269] mode=indexing
              n234 = Unbundle By Name(w269) -> ("Values"=→"JointsPosition":dbl[], "UserFramePositions"=→"UserFramePositions":T7, "World Positions"=→"World Positions":T6)  [unwired: 1 out]
            }
          }
        }
        n235 = case shown="True" w200 {
          frame False {
          }
          frame True {
            n236 = local read "Ftp"() -> (w222:refnum<k24>)
            n237 = call "GetIoState.vi"("Ftp"=w222) -> ("IO States"=w221:T14)  [unwired: 9 in, 1 out]
            n238 = for {
              tunnel: w221 -> [w246] mode=indexing
              tunnel: [w242] -> w220 mode=indexing if=w226
              tunnel: [w240] -> w219 mode=indexing if=w227
              tunnel: [w232] -> w212 mode=indexing if=w225
              tunnel: [w239] -> w218 mode=indexing if=w224
              tunnel: [w238] -> w217 mode=indexing if=w223
              tunnel: [w237] -> w216 mode=indexing if=w231
              tunnel: [w236] -> w215 mode=indexing if=w230
              tunnel: [w235] -> w214 mode=indexing if=w229
              tunnel: [w233] -> w213 mode=indexing if=w228
              n239 = Unbundle By Name(w246) -> ("PortStr"=w234:string, "Id"=w245:i32, "Name"=w244:string, "Value"=w243:bool)
              n240 = Bundle("Id"=w245, "Name"=w244, "Value"=w243) -> (w241:cluster{"Id":i32, "Name":string, "Value":bool})  [unwired: 1 in]
              n241 = case shown="\"DIN\", Default" w234 {
                tunnel: [_ _ _ _ _ _ _ w262 _] -> w242
                tunnel: w241 -> [w248 w250 w252 w254 w256 w258 w260 w262 w264]
                tunnel: [_ _ _ _ _ _ w260 _ _] -> w240
                tunnel: [_ _ _ _ _ _ _ _ w264] -> w232
                tunnel: [w248 _ _ _ _ _ _ _ _] -> w239
                tunnel: [_ w250 _ _ _ _ _ _ _] -> w238
                tunnel: [_ _ w252 _ _ _ _ _ _] -> w237
                tunnel: [_ _ _ w254 _ _ _ _ _] -> w236
                tunnel: [_ _ _ _ w256 _ _ _ _] -> w235
                tunnel: [_ _ _ _ _ w258 _ _ _] -> w233
                tunnel: [_ _ TRUE _ _ _ _ _ _] -> w231
                tunnel: [_ _ _ TRUE _ _ _ _ _] -> w230
                tunnel: [_ _ _ _ TRUE _ _ _ _] -> w229
                tunnel: [_ _ _ _ _ TRUE _ _ _] -> w228
                tunnel: [_ _ _ _ _ _ TRUE _ _] -> w227
                tunnel: [_ _ _ _ _ _ _ TRUE _] -> w226
                tunnel: [_ _ _ _ _ _ _ _ TRUE] -> w225
                tunnel: [TRUE _ _ _ _ _ _ _ _] -> w224
                tunnel: [_ TRUE _ _ _ _ _ _ _] -> w223
                frame "DOUT" {
                }
                frame "UI" {
                }
                frame "UO" {
                }
                frame "SI" {
                }
                frame "SO" {
                }
                frame "RI" {
                }
                frame "RO" {
                }
                frame "FLG" {
                }
                frame "DIN", Default {
                }
              }
            }
            "FLG" <- w220
            "RO" <- w219
            "DIN" <- w212
            "DOUT" <- w218
            "UI" <- w217
            "UO" <- w216
            "SI" <- w215
            "SO" <- w214
            "RI" <- w213
          }
        }
      }
    }
    n242 = property on="FTP warning" class="Str"("Visible"=w59) -> ()  [unwired: 2 in, 2 out]
    n243 = case shown="True" w58 {
      tunnel: [T12."Disabled and Grayed Out" ("Disabled") T12."Enabled" ("Disabled")] -> w57
      frame False {
      }
      frame True {
      }
    }
    n244 = property on="Get all errors" class="Bool"("DisabledEnum"=w57) -> ()  [unwired: 2 in, 2 out]
    n245 = property on="Get safety status" class="Bool"("DisabledEnum"=w57) -> ()  [unwired: 2 in, 2 out]
    n246 = property on="Get current position" class="Bool"("DisabledEnum"=w57) -> ()  [unwired: 2 in, 2 out]
    n247 = property on="Get numeric registers" class="Bool"("DisabledEnum"=w57) -> ()  [unwired: 2 in, 2 out]
    n248 = property on="Get IO State" class="Bool"("DisabledEnum"=w57) -> ()  [unwired: 2 in, 2 out]
    n249 = property on="Get position registers" class="Bool"("DisabledEnum"=w57) -> ()  [unwired: 2 in, 2 out]
    n250 = property on="Get string registers" class="Bool"("DisabledEnum"=w57) -> ()  [unwired: 2 in, 2 out]
    n251 = local read "Snpx"() -> (w55:refnum<k24>)
    n252 = call "SnpxIsConnected.vi"("Snpx"=w55) -> ("Connected"=w45:bool)  [unwired: 9 in, 1 out]
    "SNPX connected" <- w45
    n253 = Not(x=w45) -> (.not. x?=w56:bool)
    n254 = case shown="True" w45 {
      tunnel: [T12."Disabled and Grayed Out" ("Disabled") T12."Enabled" ("Disabled")] -> w44
      frame False {
      }
      frame True {
      }
    }
    n255 = case shown="True" w45 {
      tunnel: "Continuous read world position" -> [_ w158]
      tunnel: "Continuous read user frame position" -> [_ w157]
      tunnel: "Read numeric register" -> [_ w156]
      tunnel: "Write numeric register" -> [_ w155]
      tunnel: "Read string register" -> [_ w150]
      tunnel: "Write string register" -> [_ w149]
      tunnel: "Read position register" -> [_ w148]
      tunnel: "Write cartesian position register" -> [_ w147]
      tunnel: "Write joints position register" -> [_ w143]
      frame False {
      }
      frame True {
        n256 = case shown="True" w158 {
          frame False {
          }
          frame True {
            n257 = local read "Snpx"() -> (w188:refnum<k24>)
            n258 = call "GetWorldPosition.vi"("Snpx"=w188) -> ("UserTool"=→"UserTool":i16, "Cartesian position"=→"Cartesian position":T11, "JointsPosition"=→"JointsPosition":dbl[], "error out"=→"error out":errorcluster)  [unwired: 7 in]
          }
        }
        n259 = case shown="True" w157 {
          frame False {
          }
          frame True {
            n260 = local read "Snpx"() -> (w184:refnum<k24>)
            n261 = call "GetUserFramePosition.vi"("userFrame"="userFrame", "Snpx"=w184) -> ("UserTool"=→"UserTool":i16, "Cartesian position"=→"Cartesian position":T11, "error out"=→"error out 2":errorcluster)  [unwired: 6 in, 1 out]
          }
        }
        n262 = case shown="True" w150 {
          tunnel: "String register" -> [_ w175]
          frame False {
          }
          frame True {
            n263 = local read "Snpx"() -> (w176:refnum<k24>)
            n264 = call "ReadStringRegister.vi"("index"=w175, "Snpx"=w176) -> ("Value"=→"Value":string)  [unwired: 8 in, 1 out]
          }
        }
        n265 = case shown="True" w143 {
          tunnel: "Position register" -> [_ w160]
          tunnel: "Joints position" -> [_ w159]
          frame False {
          }
          frame True {
            n266 = local read "Snpx"() -> (w161:refnum<k24>)
            n267 = call "WriteJointPositionRegister.vi"("Value"=w159, "index"=w160, "Snpx"=w161) -> ()  [unwired: 8 in, 1 out]
          }
        }
        n268 = case shown="True" w148 {
          tunnel: "Position register" -> [_ w169]
          frame False {
          }
          frame True {
            n269 = local read "Snpx"() -> (w170:refnum<k24>)
            n270 = call "ReadPositionRegister.vi"("Snpx"=w170, "index"=w169) -> ("UserFrame"=→"UserFrame":i16, "Cartesian position"=w168:T10, "UserTool"=→"UserTool":i16, "Joint position"=w165:dbl[])  [unwired: 9 in, 1 out]
            n271 = property on="Cartesian position" class="Clust (strict)"("Value"=w168) -> ()  [unwired: 2 in, 2 out]
            n272 = property on="Joints position" class="Arr (strict)"("Value"=w165) -> ()  [unwired: 2 in, 2 out]
          }
        }
        n273 = case shown="True" w149 {
          tunnel: "String register" -> [_ w172]
          tunnel: "New value" -> [_ w171]
          frame False {
          }
          frame True {
            n274 = local read "Snpx"() -> (w173:refnum<k24>)
            n275 = call "WriteStringRegister.vi"("value"=w171, "index"=w172, "Snpx"=w173) -> ()  [unwired: 8 in, 1 out]
          }
        }
        n276 = case shown="True" w156 {
          tunnel: "Numeric register" -> [_ w181]
          frame False {
          }
          frame True {
            n277 = local read "Snpx"() -> (w182:refnum<k24>)
            n278 = call "ReadNumericRegister.vi"("index"=w181, "Snpx"=w182) -> ("Value"=→"Value":sgl)  [unwired: 8 in, 1 out]
          }
        }
        n279 = case shown="True" w147 {
          tunnel: "Cartesian position 2" -> [_ w163]
          tunnel: "Position register" -> [_ w162]
          frame False {
          }
          frame True {
            n280 = local read "Snpx"() -> (w164:refnum<k24>)
            n281 = call "WriteCartesianPositionRegister.vi"("Cartesian position"=w163, "index"=w162, "Snpx"=w164) -> ()  [unwired: 8 in, 1 out]
          }
        }
        n282 = case shown="True" w155 {
          tunnel: "New value" -> [_ w178]
          tunnel: "Numeric register" -> [_ w177]
          frame False {
          }
          frame True {
            n283 = local read "Snpx"() -> (w179:refnum<k24>)
            n284 = call "WriteNumericRegister.vi"("Value"=w178, "index"=w177, "Snpx"=w179) -> ()  [unwired: 8 in, 1 out]
          }
        }
      }
    }
    n285 = property on="SNPX warning" class="Str"("Visible"=w56) -> ()  [unwired: 2 in, 2 out]
    n286 = property on="Read string register" class="Bool"("DisabledEnum"=w44) -> ()  [unwired: 2 in, 2 out]
    n287 = property on="Write string register" class="Bool"("DisabledEnum"=w44) -> ()  [unwired: 2 in, 2 out]
    n288 = property on="Read numeric register" class="Bool"("DisabledEnum"=w44) -> ()  [unwired: 2 in, 2 out]
    n289 = property on="Write numeric register" class="Bool"("DisabledEnum"=w44) -> ()  [unwired: 2 in, 2 out]
    n290 = property on="Write joints position register" class="Bool"("DisabledEnum"=w44) -> ()  [unwired: 2 in, 2 out]
    n291 = property on="Continuous read user frame position" class="Bool (strict)"("DisabledEnum"=w44) -> ()  [unwired: 2 in, 2 out]
    n292 = property on="Write cartesian position register" class="Bool"("DisabledEnum"=w44) -> ()  [unwired: 2 in, 2 out]
    n293 = property on="Continuous read world position" class="Bool (strict)"("DisabledEnum"=w44) -> ()  [unwired: 2 in, 2 out]
    n294 = property on="Read position register" class="Bool"("DisabledEnum"=w44) -> ()  [unwired: 2 in, 2 out]
    n295 = local read "Cgtp"() -> (w43:refnum<k24>)
    n296 = call "CgtpIsEnabled.vi"("Cgtp"=w43) -> ("Enabled"=w37:bool)  [unwired: 9 in, 1 out]
    "CGTP Enabled" <- w37
    n297 = case shown="True" "Write variable as real" {
      tunnel: "Variable name" -> [_ w117]
      tunnel: "New real value" -> [_ w116]
      frame False {
      }
      frame True {
        n298 = local read "Cgtp"() -> (w118:refnum<k24>)
        n299 = call "CgtpWriteVariableAsReal.vi"("Cgtp"=w118, "varName"=w117, "value"=w116) -> ()  [unwired: 12 in, 1 out]
      }
    }
    n300 = case shown="True" w37 {
      tunnel: "Program name" -> [_ w129]
      tunnel: "Run" -> [_ w132]
      tunnel: "Abort" -> [_ w131]
      tunnel: "Pause" -> [_ w130]
      frame False {
      }
      frame True {
        n301 = case shown="True" w132 {
          tunnel: w129 -> [_ w137]
          frame False {
          }
          frame True {
            n302 = local read "Cgtp"() -> (w138:refnum<k24>)
            n303 = call "CgtpRunProgram.vi"("lineNum"=1, "progName"=w137, "Cgtp"=w138) -> ()  [unwired: 8 in, 1 out]
          }
        }
        n304 = case shown="True" w130 {
          frame False {
          }
          frame True {
            n305 = local read "Cgtp"() -> (w135:refnum<k24>)
            n306 = call "CgtpPauseAllPrograms.vi"("Cgtp"=w135) -> ()  [unwired: 10 in, 1 out]
          }
        }
        n307 = case shown="True" w131 {
          tunnel: w129 -> [_ w133]
          frame False {
          }
          frame True {
            n308 = local read "Cgtp"() -> (w134:refnum<k24>)
            n309 = call "CgtpAbortTask.vi"("progName"=w133, "Cgtp"=w134) -> ()  [unwired: 9 in, 1 out]
          }
        }
      }
    }
    n310 = case shown="True" "Write variable as integer" {
      tunnel: "Variable name" -> [_ w120]
      tunnel: "String value" -> [_ w119]
      frame False {
      }
      frame True {
        n311 = local read "Cgtp"() -> (w121:refnum<k24>)
        n312 = call "CgtpWriteVariableAsString.vi"("Cgtp"=w121, "varName"=w120, "value"=w119) -> ()  [unwired: 12 in, 1 out]
      }
    }
    n313 = case shown="True" "Write variable as string" {
      tunnel: "Variable name" -> [_ w123]
      tunnel: "New integer value" -> [_ w122]
      frame False {
      }
      frame True {
        n314 = local read "Cgtp"() -> (w124:refnum<k24>)
        n315 = call "CgtpWriteVariableAsInteger.vi"("Cgtp"=w124, "varName"=w123, "value"=w122) -> ()  [unwired: 12 in, 1 out]
      }
    }
    n316 = case shown="True" "Read variable" {
      tunnel: "Variable name" -> [_ w127]
      frame False {
      }
      frame True {
        n317 = local read "Cgtp"() -> (w128:refnum<k24>)
        n318 = call "CgtpReadVariableAsString.vi"("varName"=w127, "Cgtp"=w128) -> ("String Value"=w126:string, "error out"=w125:errorcluster)  [unwired: 8 in]
        n319 = property on="String value" class="Str"(error in=w125, "Value"=w126) -> ()  [unwired: 1 in, 2 out]
      }
    }
    n320 = Not(x=w37) -> (.not. x?=w36:bool)
    n321 = case shown="True" w37 {
      tunnel: [T12."Disabled and Grayed Out" ("Disabled") T12."Enabled" ("Disabled")] -> w42
      frame False {
      }
      frame True {
      }
    }
    n322 = property on="CGTP warning" class="Str"("Visible"=w36) -> ()  [unwired: 2 in, 2 out]
    n323 = property on="Pause" class="Bool"("DisabledEnum"=w42) -> ()  [unwired: 2 in, 2 out]
    n324 = property on="Abort" class="Bool"("DisabledEnum"=w42) -> ()  [unwired: 2 in, 2 out]
    n325 = property on="Run" class="Bool"("DisabledEnum"=w42) -> ()  [unwired: 2 in, 2 out]
  }
  "TelnetError" <- "" ("ErrorText")
  "TelnetSucceed" <- FALSE ("Succeed")
  "KclCommand" <- "" ("KclCommand")
  "Telnet warning" <- "Telnet is not connected\nPlease connect to use this panel" ("Telnet warning")
  "FTP warning" <- "FTP is not connected\nPlease connect to use this panel" ("FTP warning")
  "SNPX warning" <- "SNPX is not connected\nPlease connect to use this panel" ("FTP warning")
  "CGTP warning" <- "CGTP is not connected\nPlease connect to use this panel" ("Telnet warning 2")
